vi "בדיקת זמן ניתוק הממסר 4.vi"(7 "resultUserPrompt":bool, 8 "error":errorcluster, 11 "Path for Log":path) -> (0 "error out":errorcluster, 1 "בטוח כן/לא":bool, 2 "בדיקת זמן ניתוק הממסר":dbl)   [LabVIEW 2014]
uses:
  <instrlib>/niDMM/nidmm.llb/niDMM Function.ctl
  <instrlib>/niDMM/nidmm.llb/niDMM Resolution in Digits.ctl
  <vilib>/DAQmx/create/channels.llb/DAQmx Create Channel (DO-Digital Output).vi
  <vilib>/DAQmx/write.llb/DAQmx Write (Digital Bool 1Line 1Point).vi
  <instrlib>/niDMM/nidmm.llb/niDMM Configure Measurement Digits.vi
panel:
  in  "התחל":bool
  # "Right-Click to\nexplain error"
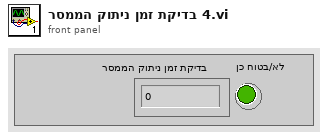
[diagram p1: front panel]
types:
  T1 = enum32{"Invalid", "Standard", "Closed", "Hidden", "Minimized", "Maximized"}
  T2 = typedef "niDMM Function.ctl" = enum16{"DC Volts", "AC Volts", "DC Current", "AC Current", "2-wire Resistance", "4-wire Resistance", "Diode", "Frequency", "Period", "AC Volts DC Coupled", "Capacitance", "Inductance", "Temperature"}
  T3 = typedef "niDMM Resolution in Digits.ctl" = dbl
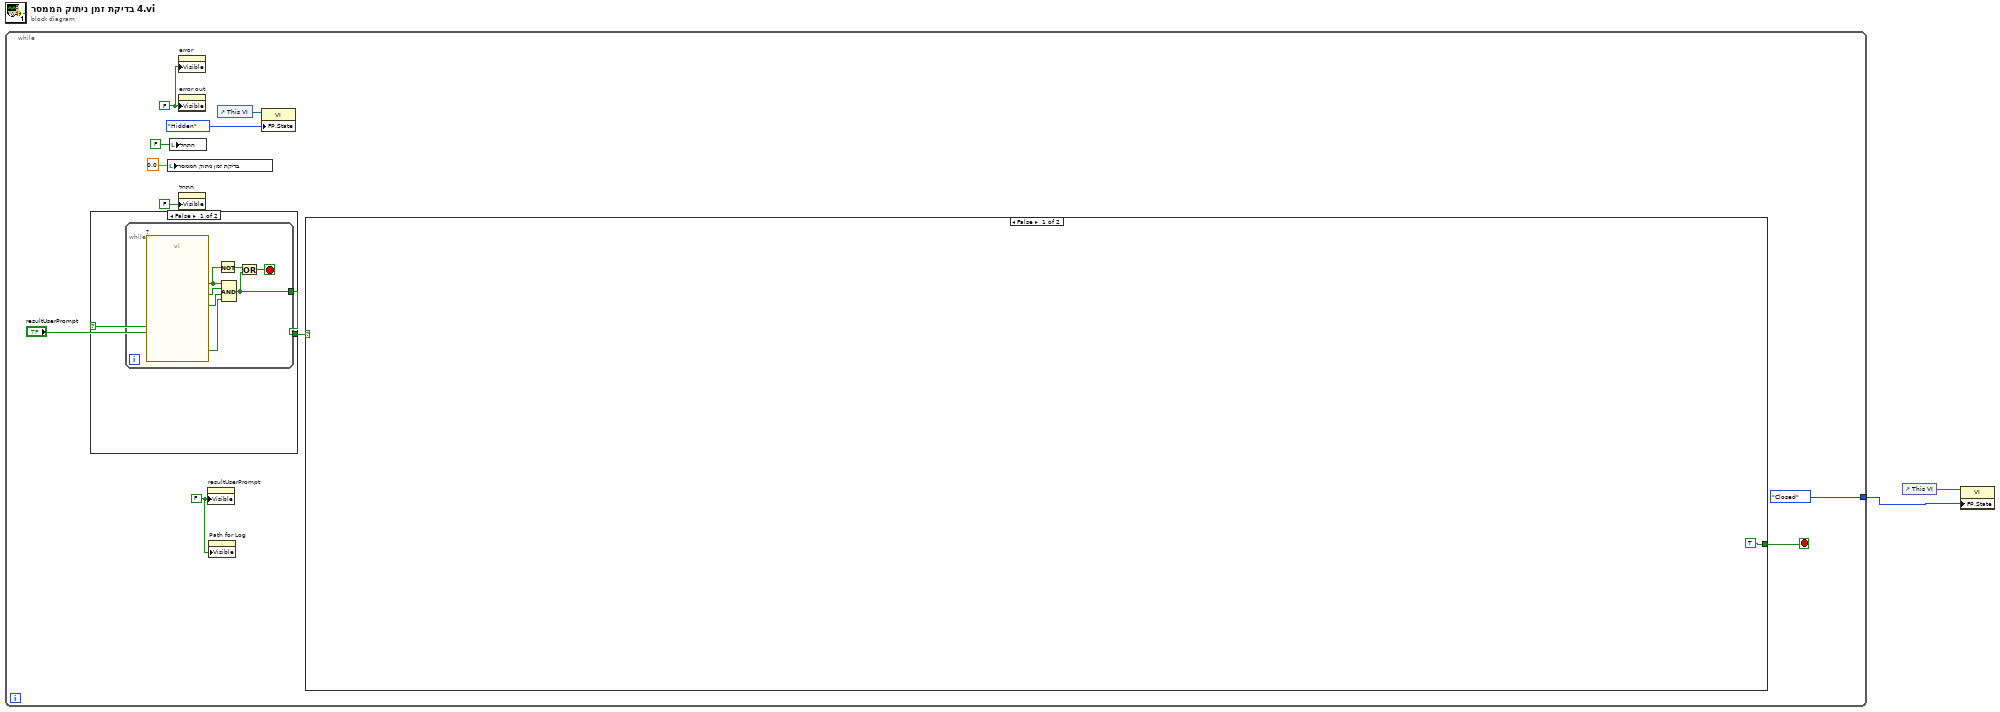
[diagram p0: block diagram]
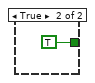
[diagram p2: hidden frame]
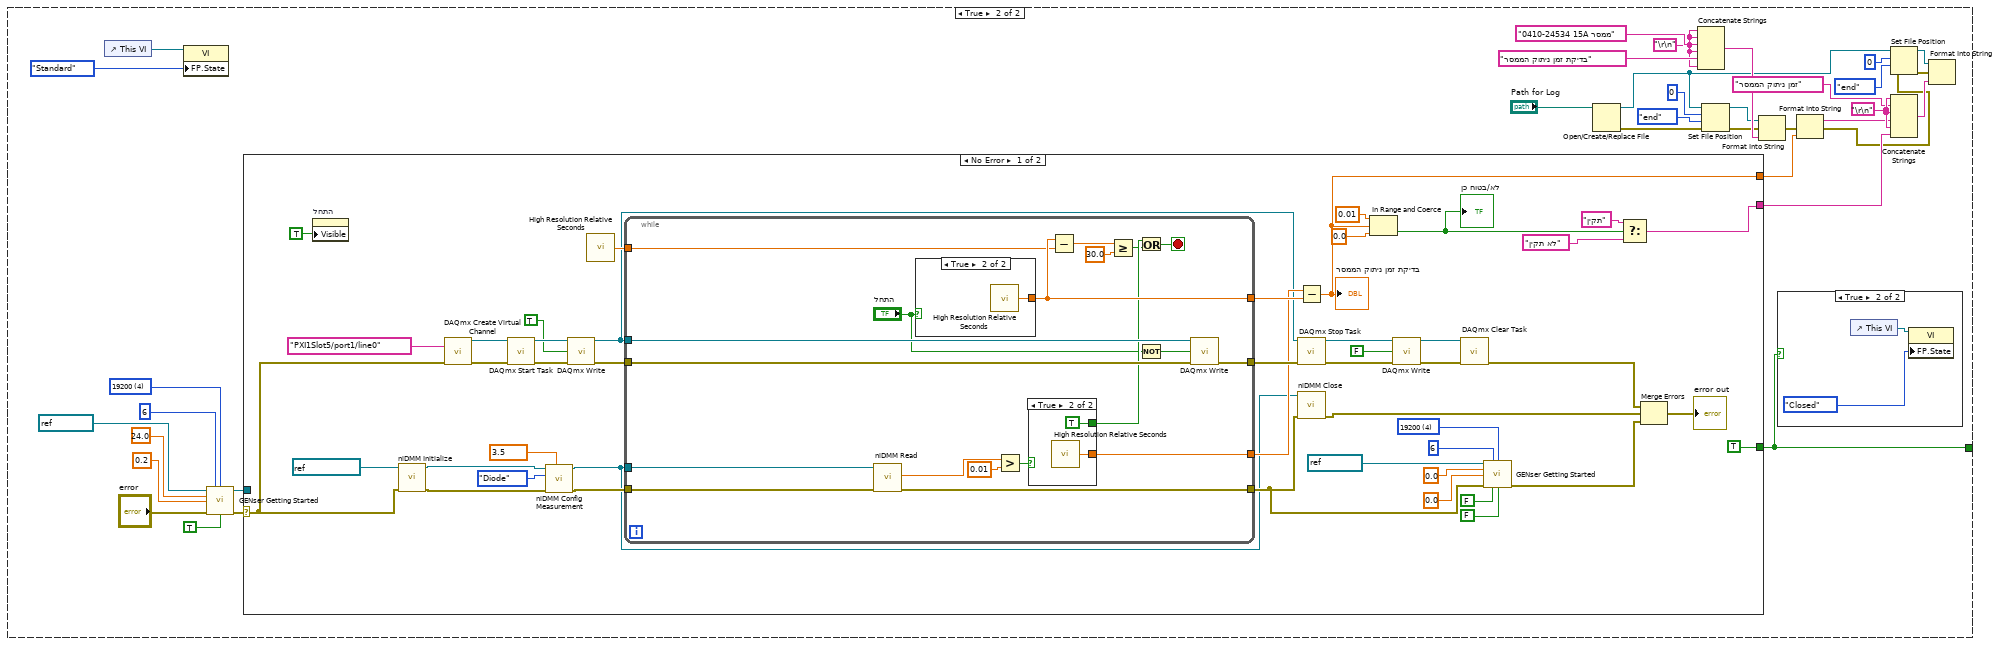
[diagram p3: hidden frame]
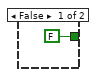
[diagram p5: hidden frame]
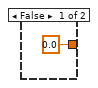
[diagram p6: hidden frame]
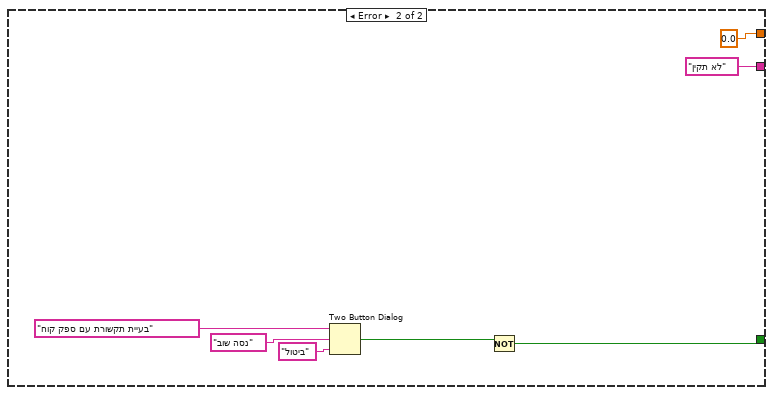
[diagram p7: hidden frame]
diagram:
  n1 = while {
    tunnel: [T1."Closed" ("Front Panel Window:State")] -> w1
    stop <- w4 stop-if-true
    w5 = FALSE ("Visible")
    w12 = FALSE ("Visible")
    n2 = case shown="False" "resultUserPrompt" {
      tunnel: [w14 TRUE] -> w13
      frame False {
        n3 = while {
          tunnel: [w15] -> w14
          stop <- w18 stop-if-true
          n4 = call "?"() -> ("הדקי הרב מודד"=w19:bool, "(מגע שלילי (מעטפת"=w20:bool, "A מגע חיובי"=w21:bool, "OK"=w17:bool)  [unwired: 15 in, 1 out]
          n5 = Not(x=w17) -> (.not. x?=w16:bool)
          n6 = Compound Arithmetic op=AND(w17, w21, w20, w19) -> (w15:bool)
          n7 = Or(x=w16, y=w15) -> (x .or. y?=w18:bool)
        }
      }
      frame True {
      }
    }
    n8 = local write "בדיקת זמן ניתוק הממסר"(0.0 ("זמן ניתוק הממסר")) -> ()
    n9 = local write "התחל"(FALSE ("זמן ניתוק הממסר בטווח כן /לא")) -> ()
    n10 = property on="error" class="Clust (strict)"("Visible"=w12) -> ()  [unwired: 2 in, 2 out]
    n11 = property on="error out" class="Clust (strict)"("Visible"=w12) -> ()  [unwired: 2 in, 2 out]
    n12 = property on="התחל" class="Bool (strict)"("Visible"=FALSE) -> ()  [unwired: 2 in, 2 out]
    n13 = property on="resultUserPrompt" class="Bool (strict)"("Visible"=w5) -> ()  [unwired: 2 in, 2 out]
    n14 = property on="Path for Log" class="Path"("Visible"=w5) -> ()  [unwired: 2 in, 2 out]
    n15 = control-ref of="This VI"() -> (w11:refnum<vi>)
    n16 = property class="VI"(reference=w11, "FP.State"=T1."Hidden" ("Front Panel Window:State")) -> ()  [unwired: 1 in, 2 out]
    n17 = case shown="False" w13 {
      tunnel: [TRUE ("T button?") w24] -> w4
      frame False {
      }
      frame True {
        w33 = "\r\n"
        w41 = "\r\n"
        w55 = u16 4 items=["1200", "2400", "4800", "9600", "19200"] ("BAUD")
        n18 = control-ref of="This VI"() -> (w51:refnum<vi>)
        n19 = property class="VI"(reference=w51, "FP.State"=T1."Standard" ("Front Panel Window:State")) -> ()  [unwired: 1 in, 2 out]
        n20 = call "GENser Getting Started.vi"("VISA"=refnum<visa-resource-name> "COM6", "GEN Addr"=i16 6, "BAUD"=w55, "Voltage Limit"=24.0, "Current Limit"=0.2, "error"="error", "Output On (T)"=TRUE) -> ("VISA out"=w56:refnum<visa-resource-name>, "error out"=w48:errorcluster)  [unwired: 5 in, 2 out]
        n21 = case shown="No Error" w48 {
          selector: w48 -> [w64 _]
          tunnel: w56 -> [_ _]
          tunnel: [TRUE ("T button?") w131] -> w24
          tunnel: [w85 0.0] -> w27
          tunnel: [w81 "לא תקין"] -> w26
          frame No Error {
            w69 = T3 3.5 items=["3 1/2"=3.5, "4 1/2"=4.5, "5 1/2"=5.5, "6 1/2"=6.5, "7 1/2"=7.5] ("Resolution in Digits")
            w99 = u16 4 items=["1200", "2400", "4800", "9600", "19200"] ("BAUD")
            n22 = property on="התחל" class="Bool (strict)"("Visible"=TRUE) -> ()  [unwired: 2 in, 2 out]
            n23 = call <instrlib>:"niDMM Initialize.vi"("error in (no error)"=w64, "Instrument Descriptor"=refnum<k15> "PXI1Slot9") -> ("error out"=w66:errorcluster, "instrument handle out"=w67:refnum<k15>)  [unwired: 8 in]
            n24 = call-poly <vilib>:"DAQmx Create Virtual Channel.vi"("lines"=tag "PXI1Slot5/port1/line0", "error in"=w64) -> ("task out"=w78:refnum<k21>, "error out"=w79:errorcluster)  [unwired: 12 in]
            n25 = call <vilib>:"DAQmx Start Task.vi"("task/channels in"=w78, "error in"=w79) -> ("task out"=w75:refnum<k21>, "error out"=w74:errorcluster)  [unwired: 12 in]
            n26 = call-poly <instrlib>:"niDMM Config Measurement.vi"("Resolution in Digits"=w69, "error in (no error)"=w66, "Function"=niDMM_Function."Diode", "instrument handle"=w67) -> ("error out"=w68:errorcluster, "instrument handle out"=w63:refnum<k15>)  [unwired: 6 in]
            n27 = call-poly <vilib>:"DAQmx Write.vi"("task/channels in"=w75, "data"=TRUE, "error in"=w74) -> ("task out"=w62:refnum<k21>, "error out"=w73:errorcluster)  [unwired: 10 in, 1 out]
            n28 = call <vilib>:"High Resolution Relative Seconds.vi"() -> ("relative seconds"=w76:dbl)
            n29 = while {
              tunnel: [w120] -> w87
              tunnel: [w125] -> w86
              tunnel: [w124] -> w92
              tunnel: [w121] -> w65
              tunnel: w62 -> [w123]
              tunnel: w73 -> [w122]
              tunnel: w76 -> [w119]
              tunnel: w63 -> [w111]
              tunnel: w68 -> [w110]
              stop <- w116 stop-if-true
              n30 = call <instrlib>:"niDMM Read.vi"("error in (no error)"=w110, "instrument handle"=w111) -> ("error out"=w121:errorcluster, "Measurement"=w109:dbl)  [unwired: 7 in, 1 out]
              n31 = case shown="True" "התחל" {
                tunnel: [0.0 ("relative seconds") w130] -> w120
                frame False {
                }
                frame True {
                  n32 = call <vilib>:"High Resolution Relative Seconds.vi"() -> ("relative seconds"=w130:dbl)
                }
              }
              n33 = Greater?(x=w109, y=0.01) -> (0:w107:bool)
              n34 = case shown="True" w107 {
                tunnel: [_ w128] -> w125
                tunnel: [FALSE TRUE] -> w115
                frame False {
                }
                frame True {
                  n35 = call <vilib>:"High Resolution Relative Seconds.vi"() -> ("relative seconds"=w128:dbl)
                }
              }
              n36 = Subtract(x=w120, y=w119) -> (x-y=w118:dbl)
              n37 = Greater Or Equal?(x=w118, y=30.0) -> (x >= y?=w114:bool)
              n38 = Or(x=w115, y=w114) -> (x .or. y?=w116:bool)
              n39 = Not(x="התחל") -> (.not. x?=w113:bool)
              n40 = call-poly <vilib>:"DAQmx Write.vi"("task/channels in"=w123, "data"=w113, "error in"=w122) -> ("error out"=w124:errorcluster)  [unwired: 10 in, 2 out]
            }
            n41 = Subtract(x=w86, y=w87) -> (x-y=w85:dbl)
            "בדיקת זמן ניתוק הממסר" <- w85
            n42 = call <vilib>:"DAQmx Stop Task.vi"("task/channels in"=w62, "error in"=w92) -> ("task out"=w97:refnum<k21>, "error out"=w96:errorcluster)  [unwired: 12 in]
            n43 = call <instrlib>:"niDMM Close.vi"("error in (no error)"=w65, "instrument handle"=w63) -> ("error out"=w90:errorcluster)  [unwired: 9 in]
            n44 = In Range and Coerce(upper limit=0.01, x=w85, lower limit=0.0) -> (In Range?=w82:bool)  [unwired: 1 out]
            "בטוח כן/לא" <- w82
            n45 = call-poly <vilib>:"DAQmx Write.vi"("task/channels in"=w97, "data"=FALSE, "error in"=w96) -> ("task out"=w94:refnum<k21>, "error out"=w95:errorcluster)  [unwired: 10 in, 1 out]
            n46 = call <vilib>:"DAQmx Clear Task.vi"("task in"=w94, "error in"=w95) -> ("error out"=w91:errorcluster)  [unwired: 13 in]
            n47 = call "GENser Getting Started.vi"("VISA"=refnum<visa-resource-name> "COM6", "GEN Addr"=i16 6, "BAUD"=w99, "Voltage Limit"=0.0, "Current Limit"=0.0, "error"=w65, "Reset (T)"=FALSE ("Output On (T)"), "Output On (T)"=FALSE) -> ("error out"=w61:errorcluster)  [unwired: 4 in, 3 out]
            n48 = Select(t="תקין", s=w82, f="לא תקין") -> (s? t:f=w81:string)
            n49 = Merge Errors(w91, w90, w61) -> (→"error out":errorcluster)
          }
          frame Error {
            n50 = Two Button Dialog(message="בעיית תקשורת עם ספק קוח", 1:"ביטול" ("F button name (\"Cancel\")"), 2:"נסה שוב" ("T button name (\"OK\")")) -> (T button?=w132:bool)
            n51 = Not(x=w132) -> (.not. x?=w131:bool)
          }
        }
        n52 = Open/Create/Replace File(file path (use dialog)="Path for Log") -> (refnum out=w28:refnum<file>, error out=w29:errorcluster)  [unwired: 5 in, 1 out]
        n53 = Concatenate Strings(w41, w41, "0410-24534 15A ממסר", w41, "בדיקת זמן ניתוק הממסר", w41) -> (w45:string)
        n54 = Set File Position(offset (in bytes) (0)=i64 0, refnum=w28, from (0:start)=enum16{"start", "end", "current"}."end", error in=w29) -> (refnum out=w42:refnum<file>, error out=w40:errorcluster)
        n55 = Format Into String(initial string=w42, error in=w40, w45) -> (error out=w39:errorcluster)  [unwired: 1 in, 1 out]
        n56 = case shown="True" w24 {
          frame False {
          }
          frame True {
            n57 = control-ref of="This VI"() -> (w59:refnum<vi>)
            n58 = property class="VI"(reference=w59, "FP.State"=T1."Closed" ("Front Panel Window:State")) -> ()  [unwired: 1 in, 2 out]
          }
        }
        n59 = Format Into String(error in=w39, w27) -> (resulting string=w31:string, error out=w25:errorcluster)  [unwired: 2 in]
        n60 = Set File Position(offset (in bytes) (0)=i64 0, refnum=w28, from (0:start)=enum16{"start", "end", "current"}."end", error in=w25) -> (refnum out=w36:refnum<file>, error out=w37:errorcluster)
        n61 = Concatenate Strings(w33, "זמן ניתוק הממסר", w33, w31, w33, w26) -> (w38:string)
        n62 = Format Into String(initial string=w36, error in=w37, w38) -> ()  [unwired: 1 in, 2 out]
      }
    }
  }
  n63 = control-ref of="This VI"() -> (w2:refnum<vi>)
  n64 = property class="VI"(reference=w2, "FP.State"=w1) -> ()  [unwired: 1 in, 2 out]
